vi "Read.vi"(8 "error in (no error)":errorcluster, 11 "Local Bus_DBL":refnum<class "Local Bus_I8.lvclass">) -> (0 "error out":errorcluster, 2 "Value":i8, 3 "Local Bus_DBL out":refnum<class "Local Bus_I8.lvclass">)   [LabVIEW 2021, in "Local Bus_I8.lvclass"]
uses:
  Local Bus_I8.lvclass
  Local Bus_I8.lvclass/Local Bus_I8.ctl
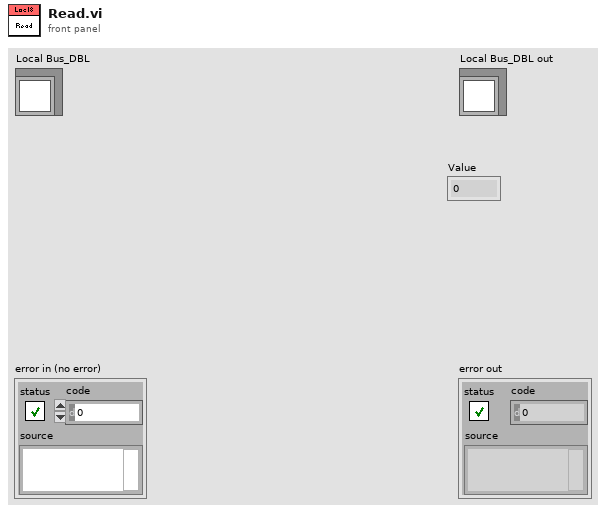
[diagram p1: front panel]
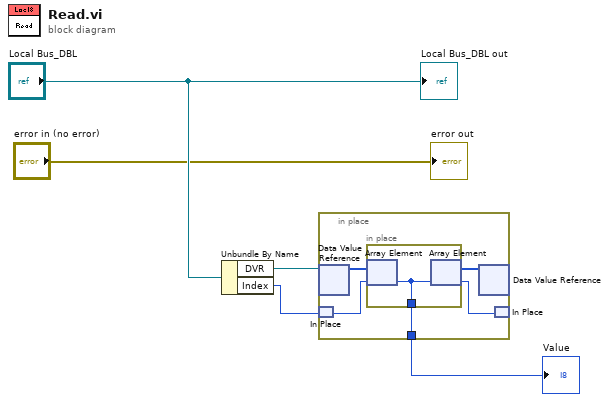
[diagram p0: block diagram]
diagram:
  n1 = Unbundle By Name("Local Bus_DBL") -> ("DVR"=w2:refnum<data-value>, "Index"=w1:i32)
  n2 = in-place {
    in-place-border: [w8] -> w3
    n3 = in-place-dvr #1(w2) -> (w10:i8[])  [unwired: 1 out]
    n4 = in-place-match #2(w1) -> (w7:i32)
    n5 = in-place {
      in-place-border: [w11] -> w8
      n6 = in-place-array #3(w10, w7) -> (w11:i8)
      n7 = in-place-array #3(w11) -> (w9:i8[], w6:i32)
    }
    n8 = in-place-dvr #1(w9) -> ()  [unwired: 2 out]
    n9 = in-place-match #2(w6) -> ()  [unwired: 1 out]
  }
  "Value" <- w3
  "error out" <- "error in (no error)"
  "Local Bus_DBL out" <- "Local Bus_DBL"
